vi "CRYGraph Result Window.vi"() -> ()   [LabVIEW 2013]
uses:
  Control/CRYResult Property.ctl
  Control/CRYFlag Cluster.ctl
  SubVI/CRYData View Global.vi
  SubVI/CRYMain Sub Window Global.vi
  CRYCurveLibrary/Global/CRYCurve Library Global.vi
panel:
  in  "LoadFinish":bool
  in  "ResultListbox":i32(listbox)
  out "Verdict":bool=TRUE
  out "Event Name":string
  out "PropertyTab":string
  in  "OpenProperty":bool
  out "TotalPlot":u32
  in  "Index":i32
  out "ReportDrop":bool
  out "Test":string
  in  "Cursor":string[][](table)
  out "Cursor Ref":refnum<vi>
  out "Queue Name":string
  in  "StateOut":bool
  in  "CursorShow":bool
  out "Result Property":T1={"Show Limits"=FALSE, "Show Yield"=FALSE, "Pass/Fail"=FALSE, "Notation"=0, "Digits"=0, "Precision"=0, "Hide Traling Zeros"=FALSE, "Show vertical scroll bar"=FALSE, "Show horizontal scroll bar"=FALSE, "True"="NO ELECTRICAL SIGNAL DETECTED!\nCheck wiring and connections.", "False"="NO ELECTRICAL SIGNAL DETECTED!\nCheck wiring and connections.", "Font Size"=0, "Overall/Optional"=0} {"Precision" items=["Digits of precision", "Significant digits"]}
  out "Graph Ref":refnum<vi>
  out "Graph Number":i32
  in  "LegendShow":bool
  in  "stop":bool
  out "Legend Ref":refnum<vi>
  in  "Legend":i32(listbox) caption="Multicolumn Listbox"
  in  "GraphType":string
  out "Title Name":string
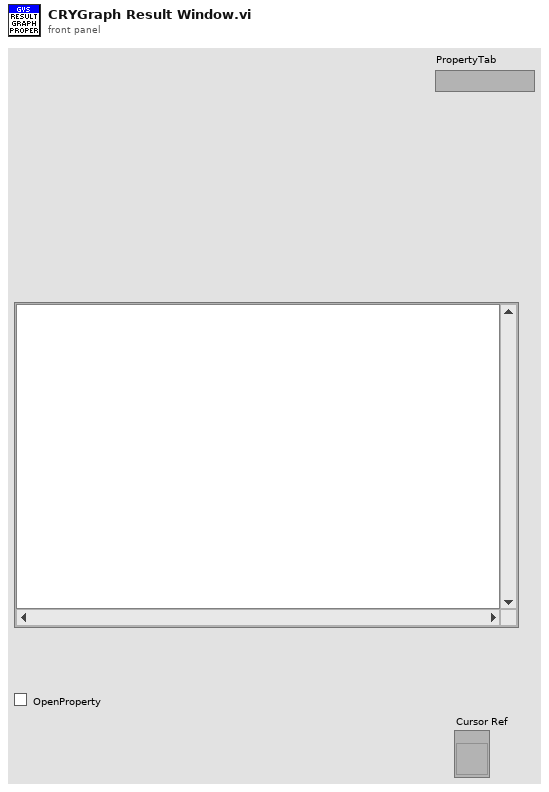
[diagram p1: front panel]
types:
  T1 = typedef "CRYResult Property.ctl" = cluster{"Show Limits":bool, "Show Yield":bool, "Pass/Fail":bool, "Notation":u16, "Digits":u16, "Precision":u16, "Hide Traling Zeros":bool, "Show vertical scroll bar":bool, "Show horizontal scroll bar":bool, "True":string, "False":string, "Font Size":u16, "Overall/Optional":u16}
  T2 = typedef "CRYGraph Event.ctl" = cluster{"EvenName":string, "TitleName":string, "GraphName":string, "GraphType":string, "Data":variant, "Queue Name":string, "DataView Number":i32}
  T3 = typedef "CRYFlag Cluster.ctl" = cluster{"LegendShow":bool, "CellClick":bool, "Total Number":bool, "ScaleFitX":bool, "ScaleFitY":bool, "MapModeX":u8, "MapModeY":u8, "CursorShow":bool, "MagnitudeShow":bool, "PreviewShow":bool, "CursorEnabled":bool, "IntensityShow":bool, "PaletteShow":bool, "PhaseShow":bool, "XYShow":bool, "FrequencyShow":bool, "LegendVScrollShow":bool, "FrequencyVScrollShow":bool}
  T4 = enum16{"Curves", "Values", "Results", "WFM", "Others"}
  T5 = typedef "LVPoint32TypeDef.ctl" = cluster{"Horizontal":i32, "Vertical":i32}
  T6 = typedef "LVRowAndColumnTypeDef.ctl" = cluster{"Row":i32, "Column":i32}
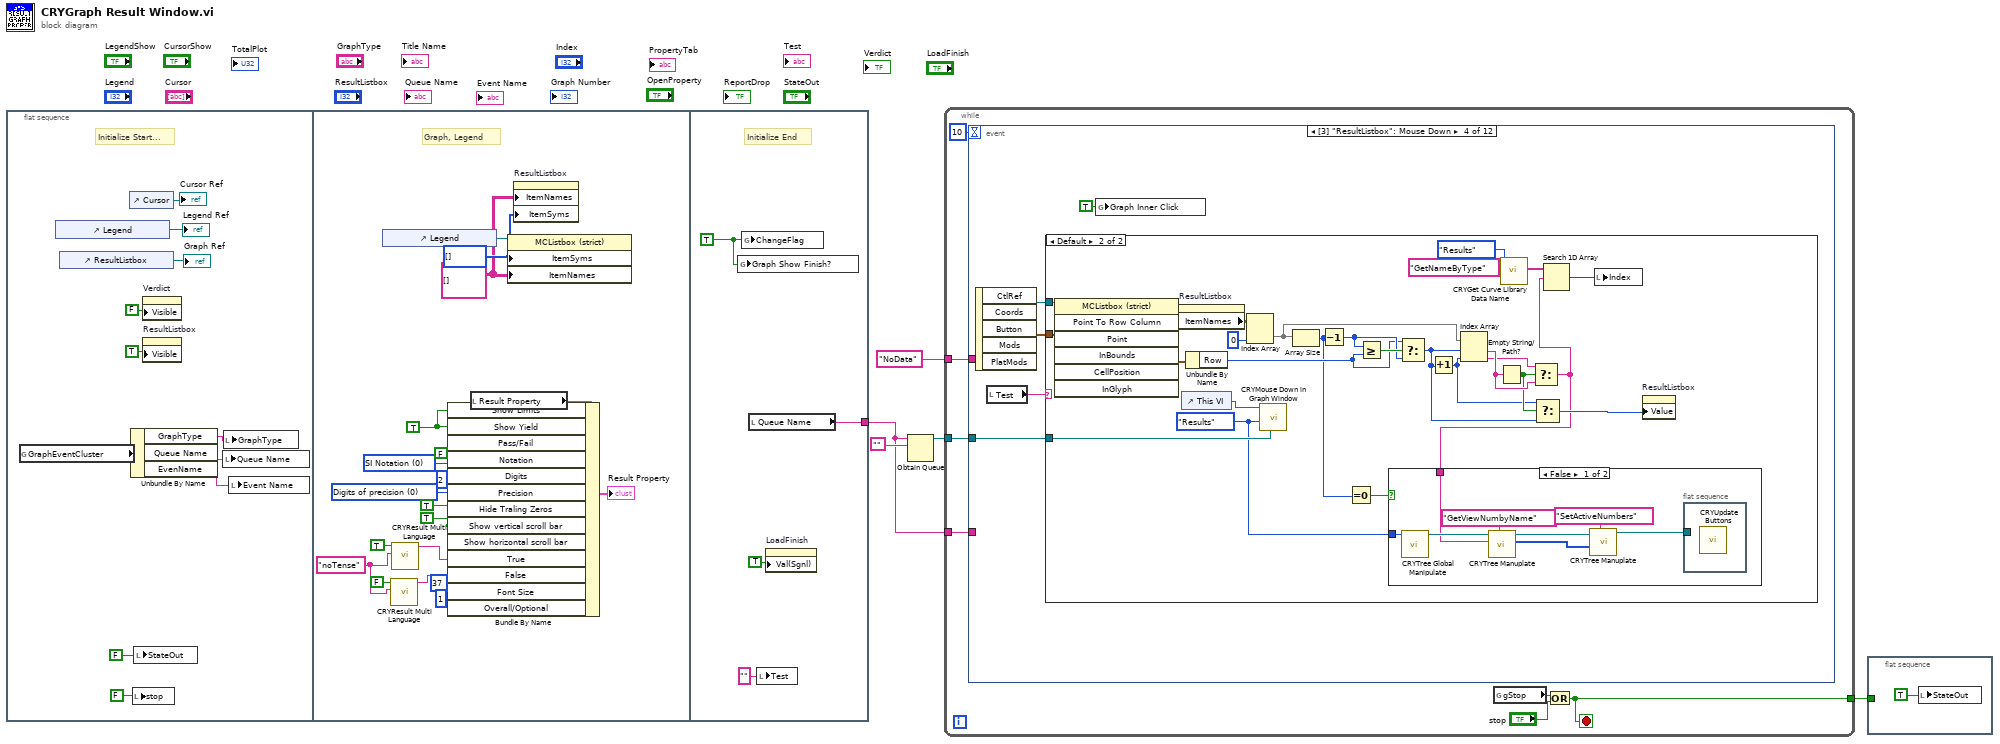
[diagram p0: block diagram]
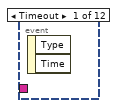
[diagram p2: hidden frame]
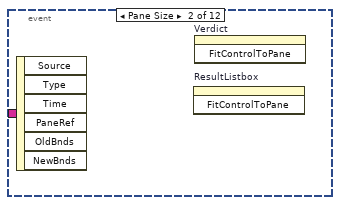
[diagram p3: hidden frame]
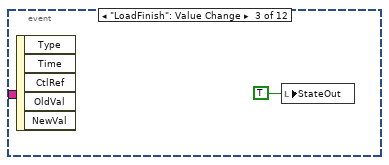
[diagram p4: hidden frame]
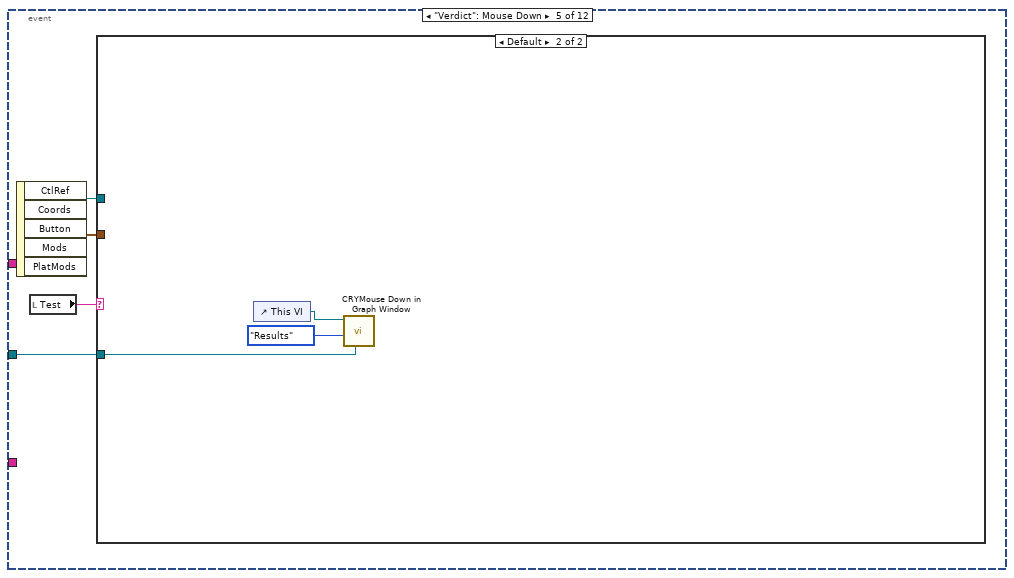
[diagram p7: hidden frame]
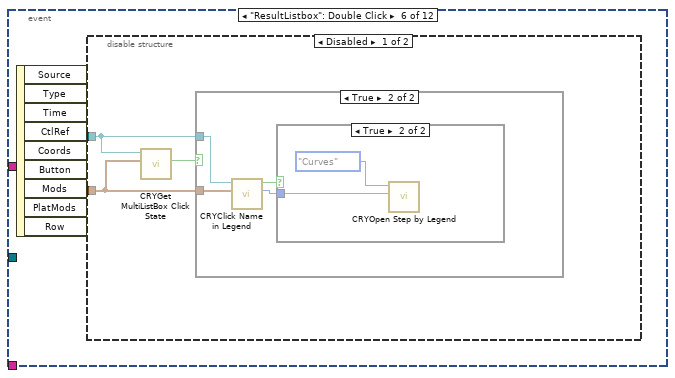
[diagram p9: hidden frame]
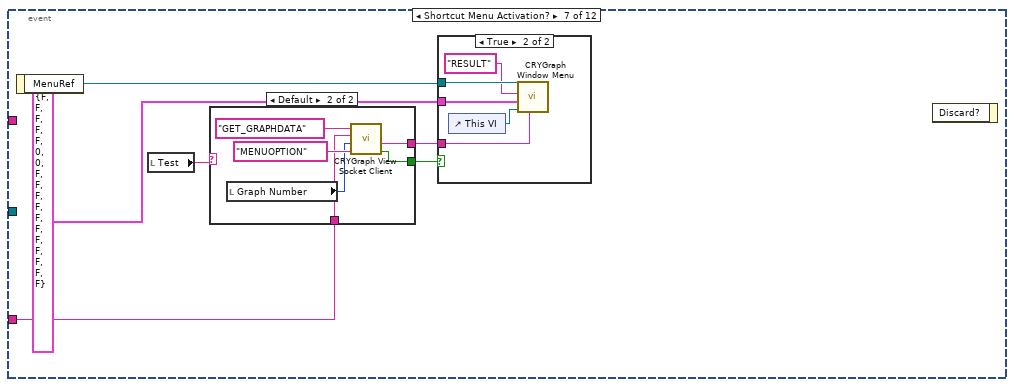
[diagram p13: hidden frame]
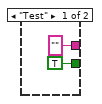
[diagram p14: hidden frame]
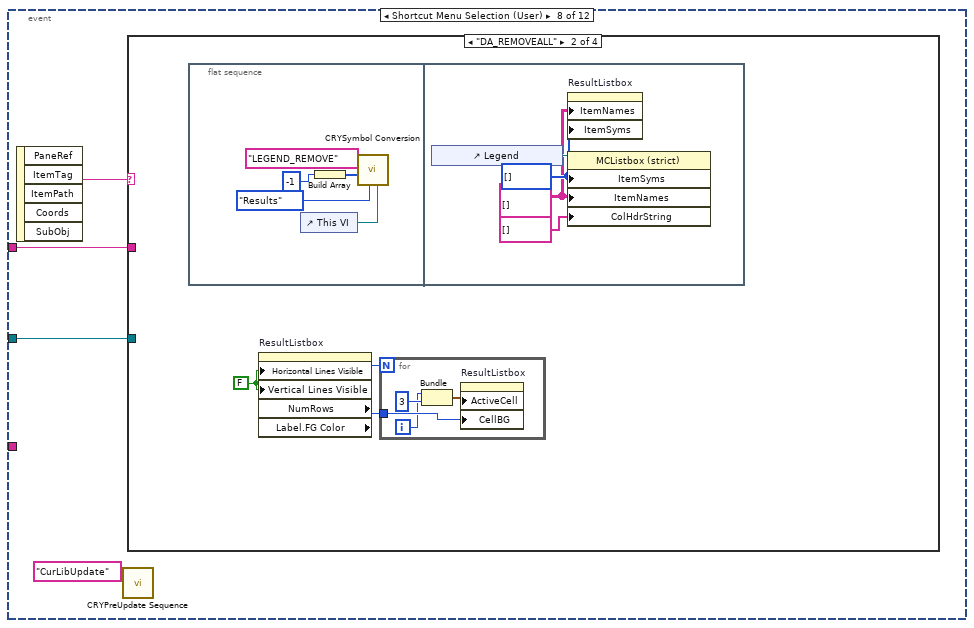
[diagram p16: hidden frame]
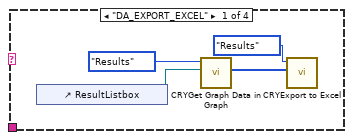
[diagram p17: hidden frame]
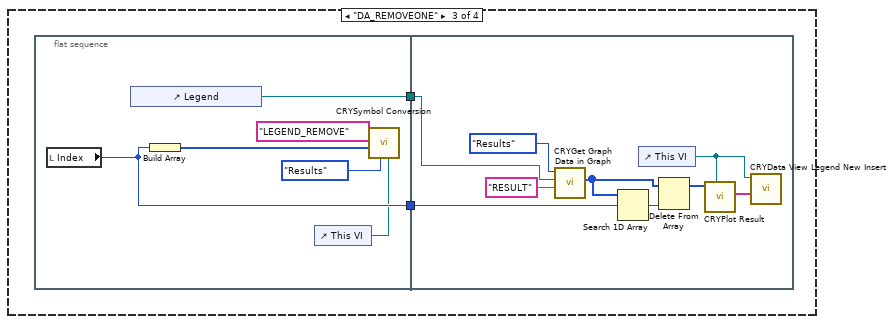
[diagram p18: hidden frame]
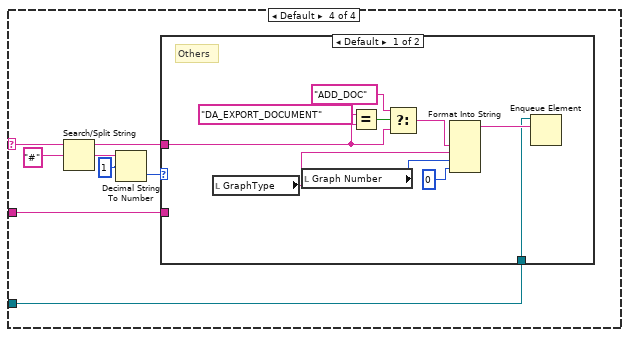
[diagram p19: hidden frame]
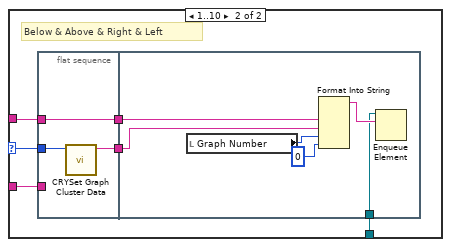
[diagram p20: hidden frame]
diagram:
  n1 = flat-sequence {
    tunnel: [w37] -> w1
    frame #0 {
      # "Initialize Start..."
      n2 = global read "CRYData View Global.vi" "GraphEventCluster"() -> (w10:T2)
      n3 = control-ref of="Legend"() -> (→"Legend Ref":refnum<vi>)
      n4 = control-ref of="ResultListbox"() -> (→"Graph Ref":refnum<vi>)
      n5 = control-ref of="Cursor"() -> (→"Cursor Ref":refnum<vi>)
      n6 = Unbundle By Name(w10) -> ("GraphType"=w9:string, "Queue Name"=w11:string, "EvenName"=w8:string)
      n7 = local write "stop"(FALSE ("stop")) -> ()
      n8 = local write "StateOut"(FALSE ("StateOut")) -> ()
      n9 = property on="Verdict" class="Bool (strict)"("Visible"=FALSE) -> ()  [unwired: 2 in, 2 out]
      n10 = property on="ResultListbox" class="MCListbox (strict)"("Visible"=TRUE) -> ()  [unwired: 2 in, 2 out]
      n11 = local write "Queue Name"(w11) -> ()
      n12 = local write "GraphType"(w9) -> ()
      n13 = local write "Event Name"(w8) -> ()
    }
    frame #1 {
      w21 = "noTense" ("sOption")
      w24 = TRUE ("Show vertical scroll bar")
      w35 = u16 0 items=["Digits of precision", "Significant digits"] ("Precision")
      w34 = u16 0 items=["SI Notation", "Floating point"] ("Notation")
      w31 = TRUE ("Show Limits")
      w26 = string[][] [] ("Item Names")
      w27 = i32[] [] ("Item Symbols")
      # "Graph, Legend"
      n14 = control-ref of="Legend"() -> (w28:refnum<vi>)
      n15 = call "CRYResult Multi Language.vi"("sOption"=w21, "Verdict"=FALSE) -> ("ASCII out"=w19:string)  [unwired: 9 in]
      n16 = call "CRYResult Multi Language.vi"("sOption"=w21, "Verdict"=TRUE) -> ("ASCII out"=w20:string)  [unwired: 9 in]
      n17 = local read "Result Property"() -> (w29:T1)
      n18 = Bundle By Name(cluster=w29, "Show Limits"=w31, "Show Yield"=w31, "Pass/Fail"=FALSE ("Overall Pass/Fail"), "Notation"=w34, "Digits"=u16 2, "Precision"=w35, "Hide Traling Zeros"=TRUE, "Show vertical scroll bar"=w24, "Show horizontal scroll bar"=w24, "True"=w20, "False"=w19, "Font Size"=u16 37, "Overall/Optional"=u16 1) -> (→"Result Property":T1)
      n19 = property on="Property Node" class="MCListbox (strict)"(reference=w28, "ItemSyms"=w27, "ItemNames"=w26) -> ()  [unwired: 1 in, 2 out]
      n20 = property on="ResultListbox" class="MCListbox (strict)"("ItemNames"=w26, "ItemSyms"=w27) -> ()  [unwired: 2 in, 2 out]
    }
    frame #2 {
      w39 = TRUE ("ChangeFlag")
      # "Initialize End"
      n21 = global write "CRYData View Global.vi" "Graph Show Finish?"(w39) -> ()
      n22 = global write "CRYData View Global.vi" "ChangeFlag"(w39) -> ()
      n23 = local read "Queue Name"() -> (w37:string)
      n24 = local write "Test"("" ("Test")) -> ()
      n25 = property on="LoadFinish" class="Bool (strict)"("Val(Sgnl)"=TRUE ("Value (Signaling)")) -> ()  [unwired: 2 in, 2 out]
    }
  }
  n26 = Obtain Queue(name (unnamed)=w1, element data type="") -> (queue out=w4:refnum<queue>)  [unwired: 3 in, 2 out]
  n27 = while {
    tunnel: w4 -> [w46]
    tunnel: "NoData" ("input 2") -> [w43]
    tunnel: w1 -> [w41]
    tunnel: [w40] -> w2
    stop <- w40 stop-if-true
    n28 = event shown="[3] \"ResultListbox\": Mouse Down" {
      selector: _ -> [_ _ _ _ _ _ _ _ _ _ _ _]
      dyn-events: _ -> [_ _ _ _ _ _ _ _ _ _ _ _]
      timeout: 10 -> [_ _ _ _ _ _ _ _ _ _ _ _]
      tunnel: w46 -> [_ _ _ w50 w87 _ _ w123 _ w207 w210 _]
      tunnel: w43 -> [_ _ _ _ _ _ _ w125 _ _ _ _]
      tunnel: w41 -> [_ _ _ _ _ _ w105 _ _ _ _ _]
      event Timeout {
        n29 = event-data() -> ()  [unwired: 3 out]
      }
      event Pane Size {
        n30 = event-data() -> ()  [unwired: 7 out]
        n31 = invoke on="ResultListbox" class="MCListbox (strict)" method="FitControlToPane"() -> ()  [unwired: 3 in, 3 out]
        n32 = invoke on="Verdict" class="Bool (strict)" method="FitControlToPane"() -> ()  [unwired: 3 in, 3 out]
      }
      event "LoadFinish": Value Change {
        n33 = event-data() -> ()  [unwired: 6 out]
        n34 = local write "StateOut"(TRUE ("StateOut")) -> ()
      }
      event "ResultListbox": Mouse Down {
        n35 = event-data() -> ("CtlRef"=w52:refnum<vi>, "Coords"=w51:T5)  [unwired: 4 out]
        n36 = local read "Test"() -> (w49:string)
        n37 = case shown="Default" w49 {
          tunnel: w52 -> [_ w77]
          tunnel: w51 -> [_ w76]
          tunnel: w50 -> [_ w75]
          frame "Test" {
          }
          frame Default {
            w55 = enum16{"Curves", "Values", "Results", "WFM"}."Results" ("Type")
            n38 = invoke class="MCListbox (strict)" method="Point To Row Column"(reference=w77, "Point"=w76) -> ("CellPosition"=w74:T6)  [unwired: 5 in, 6 out]
            n39 = property on="ResultListbox" class="MCListbox (strict)"() -> ("ItemNames"=w73:string[][])  [unwired: 2 in, 2 out]
            n40 = control-ref of="This VI"() -> (w61:refnum<vi>)
            n41 = Unbundle By Name(w74) -> ("Row"=w70:i32)
            n42 = Index Array(array=w73, index (col)=0 ("disabled index (col)")) -> (element=w69:string[])  [unwired: 1 in]
            n43 = call "CRYMouse Down in Graph Window.vi"("Queue"=w75, "Selected Type"=w55, "pGraph VI In"=w61) -> ()  [unwired: 3 in, 6 out]
            n44 = Array Size(array=w69) -> (size(s)=w54:i32)
            n45 = Decrement(x=w54) -> (x-1=w71:i32)
            n46 = Equal To 0?(x=w54) -> (x = 0?=w53:bool)
            n47 = Greater Or Equal?(x=w71, y=w70) -> (x >= y?=w72:bool)
            n48 = Select(t=w70, s=w72, f=w71) -> (s? t:f=w58:i32)
            n49 = Increment(x=w58) -> (x+1=w59:i32)
            n50 = Index Array(array=w69, index #1=w58, index #2=w59) -> (element #1=w65:string, element #2=w64:string)
            n51 = Empty String/Path?(string/path=w65) -> (empty?=w60:bool)
            n52 = call "CRYGet Curve Library Data Name.vi"("sAction"="GetNameByType", "Type"=enum16{"Curves", "Values", "Results", "WFM"}."Results") -> ("sNames"=w68:string[])  [unwired: 4 in, 5 out]
            n53 = Select(t=w64, s=w60, f=w65) -> (s? t:f=w56:string)
            n54 = case shown="False" w53 {
              tunnel: w56 -> [w82 _]
              tunnel: w55 -> [w79 _]
              frame False {
                n55 = call "CRYTree Global Manipulate.vi"("Type In"=w79) -> ("Tree/Curve Tree"=w83:refnum<vi>)  [unwired: 7 in, 3 out]
                n56 = call "CRYTree Manuplate.vi"("sAction"="GetViewNumbyName", "sOption"=w82, "Tree in"=w83) -> ("nData Out"=w81:i32[], "Tree Out"=w80:refnum<vi>)  [unwired: 5 in, 2 out]
                n57 = call "CRYTree Manuplate.vi"("sAction"="SetActiveNumbers", "nData"=w81, "Tree in"=w80) -> ("Tree Out"=w78:refnum<vi>)  [unwired: 5 in, 3 out]
                n58 = flat-sequence {
                  tunnel: w78 -> [_]
                  frame #0 {
                    n59 = call "CRYUpdate Buttons.vi"() -> ()  [unwired: 12 in]
                  }
                }
              }
              frame True {
              }
            }
            n60 = Select(t=w59, s=w60, f=w58) -> (s? t:f=w57:i32)
            n61 = Search 1D Array(1D array=w68, element=w56) -> (index of element=w62:i32)  [unwired: 1 out]
            n62 = local write "Index"(w62) -> ()
            n63 = property on="ResultListbox" class="MCListbox (strict)"("Value"=w57) -> ()  [unwired: 2 in, 2 out]
          }
        }
        n64 = global write "CRYCurve Library Global.vi" "Graph Inner Click"(TRUE ("Graph Inner Click")) -> ()
      }
      event "Verdict": Mouse Down {
        n65 = event-data() -> ("CtlRef"=w89:refnum<vi>, "Coords"=w88:T5)  [unwired: 4 out]
        n66 = local read "Test"() -> (w86:string)
        n67 = case shown="Default" w86 {
          tunnel: w89 -> [_ _]
          tunnel: w88 -> [_ _]
          tunnel: w87 -> [_ w92]
          frame "Test" {
          }
          frame Default {
            n68 = control-ref of="This VI"() -> (w90:refnum<vi>)
            n69 = call "CRYMouse Down in Graph Window.vi"("Queue"=w92, "Selected Type"=enum16{"Curves", "Values", "Results", "WFM"}."Results" ("Type"), "pGraph VI In"=w90) -> ()  [unwired: 3 in, 6 out]
          }
        }
      }
      event "ResultListbox": Double Click {
        n70 = event-data() -> ("CtlRef"=w94:refnum<vi>, "Coords"=w93:T5)  [unwired: 8 out]
        n71 = disable-structure shown="Disabled" {
          disable-tunnel: w94 -> [w96 _]
          disable-tunnel: w93 -> [w95 _]
          frame Disabled {
            n72 = call "CRYGet MultiListBox Click State.vi"("Coords"=w95, "MultiList Box Ref In"=w96) -> ("State"=w97:bool)  [unwired: 6 in, 3 out]
            n73 = case shown="True" w97 {
              tunnel: w95 -> [_ w100]
              tunnel: w96 -> [_ w101]
              frame False {
              }
              frame True {
                n74 = call "CRYClick Name in Legend.vi"("Mouse Point"=w100, "MCListbox Ref In"=w101) -> ("Active Row"=w98:i32, "Click State?"=w99:bool)  [unwired: 8 in]
                n75 = case shown="True" w99 {
                  tunnel: w98 -> [_ w103]
                  frame False {
                  }
                  frame True {
                    n76 = call "CRYOpen Step by Legend.vi"("MCListbox Ref In"=w103, "Type"=enum16{"Curves", "Values", "Results", "WFM"}."Curves" ("Type In")) -> ()  [unwired: 10 in]
                  }
                }
              }
            }
          }
          frame Enabled {
          }
        }
      }
      event Shortcut Menu Activation? {
        n77 = event-data() -> ("MenuRef"=w106:refnum<k9>)  [unwired: 1 out]
        n78 = local read "Test"() -> (w104:string)
        n79 = case shown="Default" w104 {
          tunnel: ["" ("sData Out") w115] -> w109
          tunnel: [TRUE ("bResult Out") w114] -> w108
          tunnel: w105 -> [_ w113]
          frame "Test" {
          }
          frame Default {
            n80 = local read "Graph Number"() -> (w112:i32)
            n81 = call "CRYGraph View Socket Client.vi"("sOption"="MENUOPTION", "nData"=w112, "sData"=w113, "sAction"="GET_GRAPHDATA") -> ("bResult Out"=w114:bool, "sData Out"=w115:string)  [unwired: 4 in, 2 out]
          }
        }
        n82 = case shown="True" w108 {
          tunnel: w106 -> [_ w122]
          tunnel: T3 {"LegendShow"=FALSE, "CellClick"=FALSE, "Total Number"=FALSE, "ScaleFitX"=FALSE, "ScaleFitY"=FALSE, "MapModeX"=0, "MapModeY"=0, "CursorShow"=FALSE, "MagnitudeShow"=FALSE, "PreviewShow"=FALSE, "CursorEnabled"=FALSE, "IntensityShow"=FALSE, "PaletteShow"=FALSE, "PhaseShow"=FALSE, "XYShow"=FALSE, "FrequencyShow"=FALSE, "LegendVScrollShow"=FALSE, "FrequencyVScrollShow"=FALSE} ("Flag Cluster") -> [_ w120]
          tunnel: w109 -> [_ w119]
          frame False {
          }
          frame True {
            n83 = control-ref of="This VI"() -> (w118:refnum<vi>)
            n84 = call "CRYGraph Window Menu.vi"("MenuOption"=w119, "pGraph VI"=w118, "Flag Cluster"=w120, "Type"="RESULT", "Runtime Menu Ref In"=w122) -> ()  [unwired: 7 out]
          }
        }
        n85 = event-data() -> ()  [unwired: 1 in, 2 out]
      }
      event Shortcut Menu Selection (User) {
        n86 = event-data() -> ("ItemTag"=w126:string)  [unwired: 5 out]
        n87 = call "CRYPreUpdate Sequence.vi"("EventName"="CurLibUpdate") -> ()  [unwired: 15 in]
        n88 = case shown="\"DA_REMOVEALL\"" w126 {
          selector: w126 -> [_ _ _ w166]
          tunnel: w125 -> [_ _ _ w165]
          tunnel: w123 -> [_ _ _ w164]
          frame "DA_EXPORT_EXCEL" {
            n89 = control-ref of="ResultListbox"() -> (w128:refnum<vi>)
            n90 = call "CRYGet Graph Data in Graph.vi"("Legend Refnum"=w128, "Type In"=enum16{"Curves", "Values", "Results", "WFM"}."Results" ("Type")) -> ("Rows"=w127:i32[])  [unwired: 2 in, 7 out]
            n91 = call "CRYExport to Excel.vi"("Rows"=w127, "Type"=T4."Results") -> ()  [unwired: 2 in, 8 out]
          }
          frame "DA_REMOVEALL" {
            w132 = FALSE ("Visible Items:Horizontal Lines Visible")
            n92 = flat-sequence {
              frame #0 {
                n93 = control-ref of="This VI"() -> (w139:refnum<vi>)
                n94 = Build Array(-1 ("nData")) -> (w141:i32[])
                n95 = call "CRYSymbol Conversion.vi"("pGraph VI"=w139, "CurLib Tab Type"=enum16{"Curves", "Values", "Results", "WFM"}."Results", "nDatas"=w141, "sActin"="LEGEND_REMOVE") -> ()  [unwired: 8 in]
              }
              frame #1 {
                w143 = string[][] [] ("Item Names")
                w144 = i32[] [] ("Item Symbols")
                n96 = control-ref of="Legend"() -> (w146:refnum<vi>)
                n97 = property on="ResultListbox" class="MCListbox (strict)"("ItemNames"=w143, "ItemSyms"=w144) -> ()  [unwired: 2 in, 2 out]
                n98 = property on="Property Node" class="MCListbox (strict)"(reference=w146, "ItemSyms"=w144, "ItemNames"=w143, "ColHdrString"=string[] [] ("Column Header Strings[]")) -> ()  [unwired: 1 in, 2 out]
              }
            }
            n99 = property on="ResultListbox" class="MCListbox (strict)"("Horizontal Lines Visible"=w132, "Vertical Lines Visible"=w132) -> ("NumRows"=w131:u32, "Label.FG Color"=w133:u32)  [unwired: 2 in, 2 out]
            n100 = for {
              N: w131 -> [_]
              tunnel: w133 -> [w136]
              i -> [w134]
              n101 = Bundle(w134, 3) -> (w137:cluster{i32, i32})  [unwired: 1 out]
              n102 = property on="ResultListbox" class="MCListbox (strict)"("ActiveCell"=w137, "CellBG"=w136) -> ()  [unwired: 2 in, 2 out]
            }
          }
          frame "DA_REMOVEONE" {
            n103 = flat-sequence {
              tunnel: [w153] -> w148
              tunnel: [w150] -> w147
              tunnel: w148 -> [w162]
              tunnel: w147 -> [w155]
              frame #0 {
                n104 = local read "Index"() -> (w153:i32)
                n105 = control-ref of="Legend"() -> (w150:refnum<vi>)
                n106 = Build Array(w153) -> (w151:i32[])
                n107 = control-ref of="This VI"() -> (w152:refnum<vi>)
                n108 = call "CRYSymbol Conversion.vi"("pGraph VI"=w152, "CurLib Tab Type"=enum16{"Curves", "Values", "Results", "WFM"}."Results" ("Type In"), "nDatas"=w151, "sActin"="LEGEND_REMOVE") -> ()  [unwired: 8 in]
              }
              frame #1 {
                n109 = call "CRYGet Graph Data in Graph.vi"("Graph Type"="RESULT", "Legend Refnum"=w155, "Type In"=enum16{"Curves", "Values", "Results", "WFM"}."Results") -> ("Rows"=w159:i32[])  [unwired: 1 in, 7 out]
                n110 = Search 1D Array(1D array=w159, element=w162) -> (index of element=w160:i32)  [unwired: 1 in]
                n111 = control-ref of="This VI"() -> (w156:refnum<vi>)
                n112 = Delete From Array(array=w159, index=w160) -> (array with subset deleted=w158:i32[])  [unwired: 1 in, 1 out]
                n113 = call "CRYPlot Result.vi"("pGraph VI In"=w156, "Old Rows In"=w158) -> ("Curve Name"=w157:string[])  [unwired: 4 in, 5 out]
                n114 = call "CRYData View Legend New Insert.vi"("ItemName Array"=w157, "pGraph VI In"=w156) -> ()  [unwired: 3 in, 7 out]
              }
            }
          }
          frame Default {
            n115 = Search/Split String(string=w166, search string/char (-)="#") -> (substring before match=w171:string, match + rest of string=w168:string)  [unwired: 2 out]
            n116 = Decimal String To Number(string=w168, offset=1) -> (number=w170:i32)  [unwired: 2 out]
            n117 = case shown="Default" w170 {
              selector: w170 -> [_ w185]
              tunnel: w171 -> [w174 w187]
              tunnel: w165 -> [_ w183]
              tunnel: w164 -> [w178 w182]
              frame Default {
                # "Others"
                n118 = local read "GraphType"() -> (w172:string)
                n119 = local read "Graph Number"() -> (w179:i32)
                n120 = Equal?(x="DA_EXPORT_DOCUMENT" ("y"), y=w174) -> (x = y?=w177:bool)
                n121 = Select(t="ADD_DOC", s=w177, f=w174) -> (s? t:f=w173:string)
                n122 = Format Into String(w173, w172, w179, 0 ("input 3")) -> (resulting string=w180:string)  [unwired: 3 in, 1 out]
                n123 = Enqueue Element(queue=w178, element=w180) -> ()  [unwired: 1 in, 4 out]
              }
              frame 1..10 {
                # "Below & Above & Right & Left"
                n124 = flat-sequence {
                  tunnel: w187 -> [w190]
                  tunnel: [w190] -> w186
                  tunnel: w185 -> [w189]
                  tunnel: [w188] -> w184
                  tunnel: w183 -> [_]
                  tunnel: w186 -> [w194]
                  tunnel: w184 -> [w193]
                  tunnel: w182 -> [w191]
                  frame #0 {
                    n125 = call "CRYSet Graph Cluster Data.vi"("Graph Number"=w189) -> ("DataType"=w188:string)  [unwired: 2 in, 8 out]
                  }
                  frame #1 {
                    n126 = local read "Graph Number"() -> (w192:i32)
                    n127 = Format Into String(w194, w193, w192, 0 ("input 3")) -> (resulting string=w196:string)  [unwired: 3 in, 1 out]
                    n128 = Enqueue Element(queue=w191, element=w196) -> ()  [unwired: 1 in, 4 out]
                  }
                }
              }
            }
          }
        }
      }
      event "ResultListbox": Drag Enter {
        n129 = event-data() -> ("Available Data Names"=w198:string[])  [unwired: 1 out]
        n130 = disable-structure shown="Disabled" {
          disable-tunnel: w198 -> [w200 _]
          disable-tunnel: [w199 TRUE] -> w197
          frame Disabled {
            n131 = Search 1D Array(1D array=w200, element="CRY_GRAPH_DATA") -> (index of element=w201:i32)  [unwired: 1 out]
            n132 = Not Equal?(x=w201, y=-1) -> (x != y?=w199:bool)
          }
          frame Enabled {
          }
        }
        n133 = event-data("Accepted?"=w197) -> ()  [unwired: 1 in, 1 out]
      }
      event "ResultListbox": Drop {
        n134 = event-data() -> ()  [unwired: 2 out]
        n135 = local read "Event Name"() -> (w205:string)
        n136 = control-ref of="This VI"() -> (w206:refnum<vi>)
        n137 = call "CRYDrop Data in Same Graph.vi"("pGraph VI"=w206, "Queue"=w207, "sAction"=w205) -> ("Accepted?"=w208:bool)  [unwired: 4 in, 4 out]
        n138 = event-data("Accepted?"=w208) -> ()  [unwired: 1 in, 1 out]
      }
      event "ReportDrop": Value Change {
        n139 = event-data() -> ()  [unwired: 4 out]
        n140 = local read "Event Name"() -> (w209:string)
        n141 = control-ref of="This VI"() -> (w211:refnum<vi>)
        n142 = call "CRYDrop Data in Same Graph.vi"("pGraph VI"=w211, "Queue"=w210, "sAction"=w209) -> ()  [unwired: 4 in, 5 out]
      }
      event "OpenProperty": Value Change {
        n143 = event-data() -> ()  [unwired: 4 out]
        n144 = flat-sequence {
          frame #0 {
            n145 = local read "PropertyTab"() -> (w212:string)
            n146 = control-ref of="This VI"() -> (w213:refnum<vi>)
            n147 = call "CRYGraph Property Window Main.vi"("TabName"=w212, "pGraph VI In"=w213) -> ()  [unwired: 1 in, 9 out]
          }
          frame #1 {
            n148 = local write "PropertyTab"("" ("PropertyTab")) -> ()
          }
        }
      }
    }
    n149 = global read "CRYMain Sub Window Global.vi" "gStop"() -> (w45:bool)
    n150 = Or(x=w45, y="stop") -> (x .or. y?=w40:bool)
  }
  n151 = flat-sequence {
    tunnel: w2 -> [_]
    frame #0 {
      n152 = local write "StateOut"(TRUE ("StateOut")) -> ()
    }
  }
